vi "Status Byte.vi"(8 "error in (no error)":errorcluster, 11 "VISA resource name":refnum<visa-resource-name>) -> (0 "error out":errorcluster, 1 "Status Byte Register Values":T1, 2 "Status Byte":i32, 3 "VISA resource name out":refnum<visa-resource-name>, 4 "Device Errors":cluster{"code":i32, "Text":string}[](array[cluster]))   [LabVIEW 2014, in "Stanford Research DG645 - Driver.lvlib"]
doc: "Common IEEE-488.2 Command: *STB?\nInstrument Error Check\n\nQuery the standard IEEE 488.2 serial poll status byte. The bits in the STB register have the following meaning:\n\nBit Meaning\n0 INSB - INSR summary bit\n1 BUSY - Set if delay cycle is in\n progress, otherwise cleared\n2 reserved\n3 reserved\n4 MAV - message available\n5 ESB - ESR summary bit\n6 MSS - master summary bit\n7 reserved"
uses:
  Stanford Research DG645 - Driver.lvlib
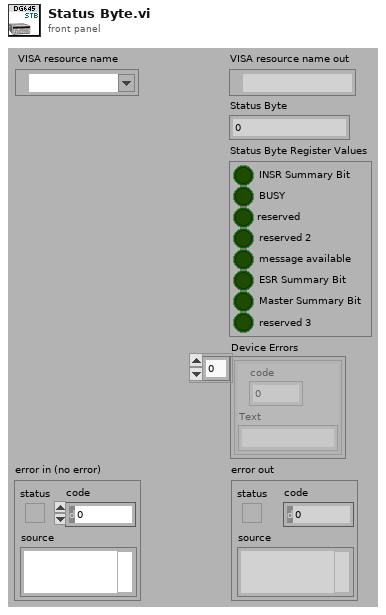
[diagram p1: front panel]
types:
  T1 = cluster{"INSR Summary Bit":bool, "BUSY":bool, "reserved":bool, "reserved 2":bool, "message available":bool, "ESR Summary Bit":bool, "Master Summary Bit":bool, "reserved 3":bool}
  T2 = cluster{"Boolean array[0]":bool, "Boolean array[1]":bool, "Boolean array[2]":bool, "Boolean array[3]":bool, "Boolean array[4]":bool, "Boolean array[5]":bool, "Boolean array[6]":bool, "Boolean array[7]":bool}
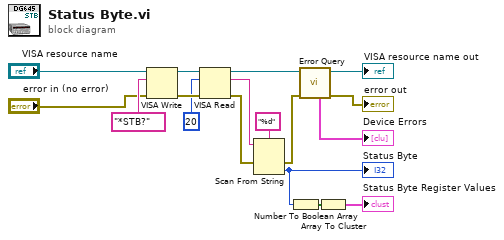
[diagram p0: block diagram]
diagram:
  n1 = VISA Write(VISA resource name="VISA resource name", write buffer="*STB?" ("Self-Test Command"), error in (no error)="error in (no error)") -> (VISA resource name out=w16:refnum<visa-resource-name>, error out=w15:errorcluster)  [unwired: 1 out]
  n2 = VISA Read(VISA resource name=w16, byte count=u32 20 ("byte count (20)"), error in (no error)=w15) -> (VISA resource name out=w5:refnum<visa-resource-name>, read buffer=w13:string, error out=w8:errorcluster)  [unwired: 1 out]
  n3 = Scan From String(format string="%d", input string=w13, error in=w8) -> (error out=w4:errorcluster, output 1=w3:i32)  [unwired: 2 in, 2 out]
  "Status Byte" <- w3
  n4 = Number To Boolean Array(number=w3) -> (Boolean array=w2:bool[])
  n5 = call "Error Query.vi"("error in (no error)"=w4, "VISA resource name"=w5) -> ("error out"=→"error out":errorcluster, "VISA resource name out"=→"VISA resource name out":refnum<visa-resource-name>, "Device Errors"=→"Device Errors":cluster{"code":i32, "Text":string}[])  [unwired: 7 in]
  n6 = Array To Cluster(array=w2) -> (cluster=→"Status Byte Register Values":T2)
